vi "apply modification.vi"(10 "vis":refnum<vi>[](array[refnum]), 11 "protection settings in":refnum<class "protection settings.lvclass">) -> (0 "error report":errorcluster[](array[cluster]), 3 "protection settings out":refnum<class "protection settings.lvclass">)   [LabVIEW 2013, in "protection settings.lvclass"]
uses:
  protection settings.lvclass
  protection settings.lvclass/protection settings.ctl
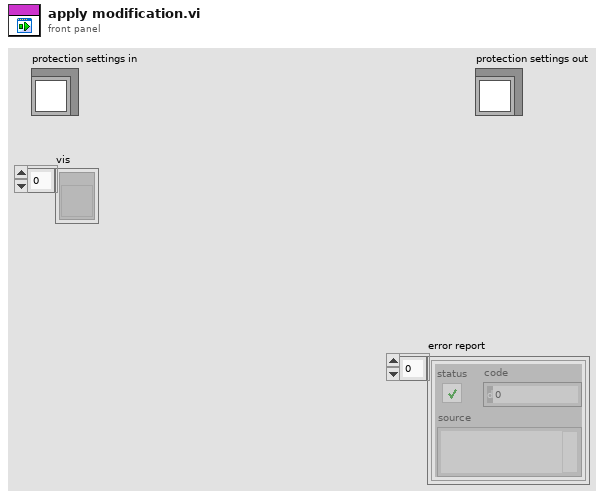
[diagram p1: front panel]
types:
  T1 = enum32{"invalid lock state", "Not Locked", "Locked (No Password)", "Password-protected"}
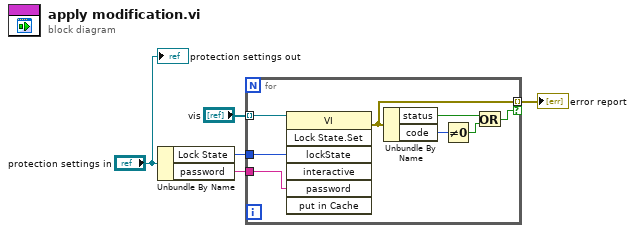
[diagram p0: block diagram]
diagram:
  n1 = Unbundle By Name("protection settings in") -> ("Lock State"=w2:T1, "password"=w3:string)
  n2 = for {
    tunnel: "vis" -> [w9] mode=indexing
    tunnel: [w8] -> w1 mode=indexing if=w10
    tunnel: w3 -> [w7]
    tunnel: w2 -> [w6]
    n3 = invoke class="VI" method="Lock State.Set"(reference=w9, "lockState"=w6, "password"=w7) -> (error out=w8:errorcluster)  [unwired: 4 in, 6 out]
    n4 = Unbundle By Name(w8) -> ("status"=w13:bool, "code"=w12:i32)
    n5 = Not Equal To 0?(x=w12) -> (x != 0?=w11:bool)
    n6 = Or(x=w13, y=w11) -> (x .or. y?=w10:bool)
  }
  "error report" <- w1
  "protection settings out" <- "protection settings in"
